vi "TCL Convert Datalog to CSV.vi"() -> ()   [LabVIEW 2010]
uses:
  <vilib>/Utility/file.llb/Write To Spreadsheet File (string).vi
panel:
  out "of":dbl
  out "file":i32
  out "file progress":dbl(slide) scale=0.0..1.0
  in  "primary key":string="EventNum"
  in  "signals":string[](array[string])=["RawSignal", "PolySignal"]
  out "error out":errorcluster
  in  "error in (no error)":errorcluster
  in  "input files (prompt)":path[](array[path])
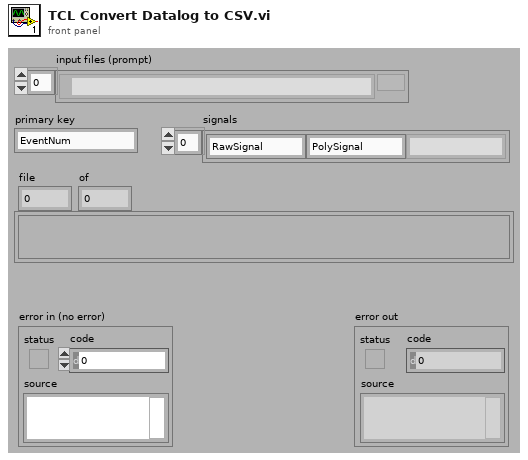
[diagram p1: front panel]
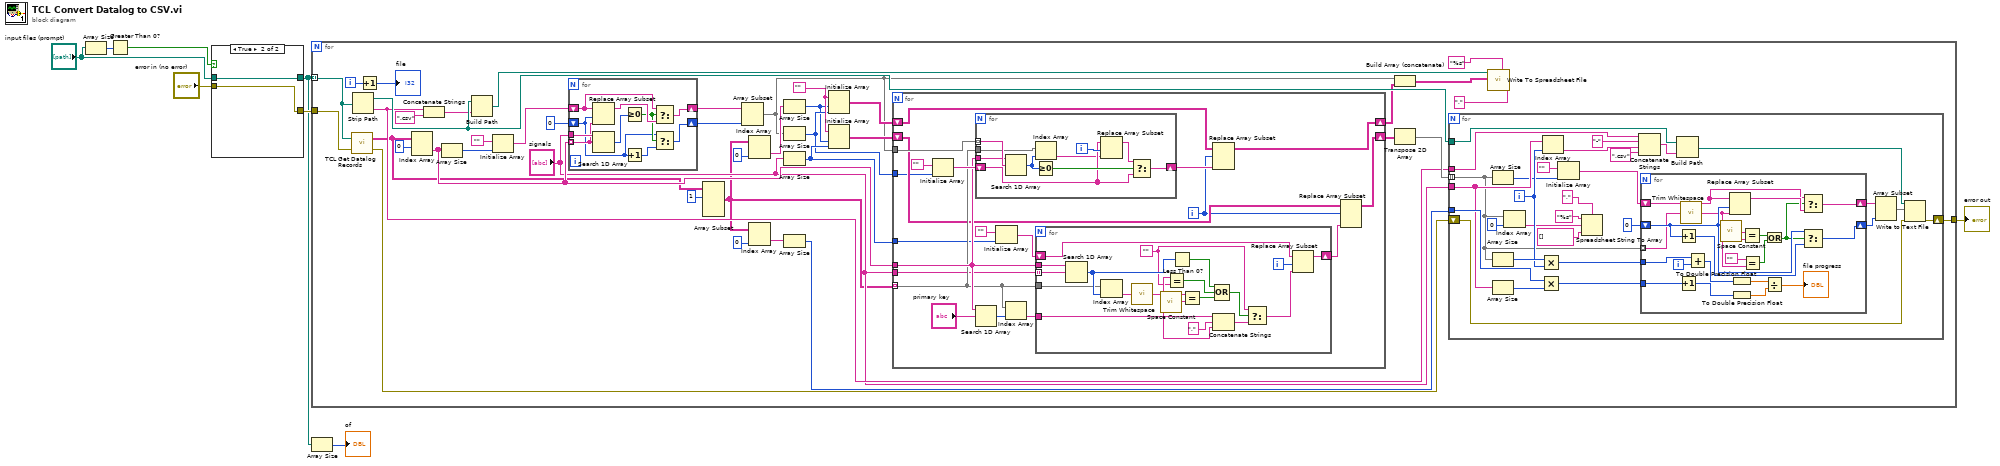
[diagram p0: block diagram]
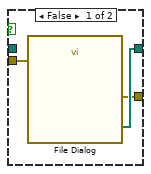
[diagram p2: hidden frame]
diagram:
  n1 = Array Size(array="input files (prompt)") -> (size(s)=w8:i32)
  n2 = Greater Than 0?(x=w8) -> (x > 0?=w7:bool)
  n3 = case shown="True" w7 {
    tunnel: [w11 w12] -> w2
    tunnel: "error in (no error)" -> [w10 w13]
    tunnel: [w9 w13] -> w5
    tunnel: "input files (prompt)" -> [_ w12]
    frame False {
      n4 = call "File Dialog"("error in"=w10) -> ("selected paths"=w11:path[], "error out"=w9:errorcluster)  [unwired: 11 in, 2 out]
    }
    frame True {
    }
  }
  n5 = for {
    tunnel: w2 -> [w50] mode=indexing
    tunnel: w5 -> [w42]
    tunnel: [w15] -> w3
    i -> [w34]
    w21 = ""
    n6 = call "TCL Get Datalog Records.vi"("error in (no error)"=w42, "event file"=w50) -> ("error out"=w14:errorcluster, "records"=w16:string[][])
    n7 = Strip Path(path=w50) -> (stripped path=w49:path, name=w46:string)
    n8 = Increment(x=w34) -> (x+1=→"file":i32)
    n9 = Index Array(array=w16, index (row)=0) -> (element=w31:string[])  [unwired: 1 in]
    n10 = Concatenate Strings(w46, ".csv" ("string")) -> (w48:string)
    n11 = Array Size(array=w31) -> (size(s)=w32:i32)
    n12 = Build Path(base path=w49, name or relative path=w48) -> (appended path=w43:path)
    n13 = Initialize Array("", w32) -> (w29:string[])
    n14 = for {
      tunnel: w31 -> [w159] mode=indexing
      tunnel: "signals" -> [w163]
      shift-right: [w161] -> w37
      shift-left: w29 -> [w158]
      shift-right: [w157] -> w28
      shift-left: 0 -> [w154]
      n15 = Replace Array Subset(array=w158, new element=w159, index=w154) -> (w160:string[])
      n16 = Search 1D Array(1D array=w163, element=w159) -> (index of element=w162:i32)  [unwired: 1 in]
      n17 = Greater Or Equal To 0?(x=w162) -> (x >= 0?=w156:bool)
      n18 = Increment(x=w154) -> (x+1=w155:i32)
      n19 = Select(t=w158, s=w156, f=w160) -> (s? t:f=w161:string[])
      n20 = Select(t=w154, s=w156, f=w155) -> (s? t:f=w157:i32)
    }
    n21 = Array Subset(array=w16, index (row)=1 ("index")) -> (w24:string[][])  [unwired: 3 in]
    n22 = Array Subset(array=w37, length=w28) -> (w20:string[])  [unwired: 1 in]
    n23 = Index Array(array=w24, index (col)=0 ("index (row)")) -> (element=w23:string[])  [unwired: 1 in]
    n24 = Index Array(array=w24, index (col)=0 ("disabled index (col)")) -> (element=w40:string[])  [unwired: 1 in]
    n25 = Array Size(array=w23) -> (size(s)=w18:i32)
    n26 = Array Size(array=w20) -> (size(s)=w19:i32)
    n27 = Array Size(array="signals") -> (size(s)=w25:i32)
    n28 = Array Size(array=w40) -> (size(s)=w36:i32)
    n29 = Initialize Array(w21, w18, w19) -> (w22:string[][])
    n30 = Initialize Array(w21, w18, w25) -> (w27:string[][])
    n31 = for {
      tunnel: w24 -> [w119] mode=indexing
      tunnel: w20 -> [w124]
      tunnel: w31 -> [w121]
      tunnel: "signals" -> [w111]
      shift-right: [w116] -> w52
      shift-left: w27 -> [w115]
      shift-right: [w113] -> w38
      shift-left: w22 -> [w114]
      tunnel: w25 -> [w109]
      tunnel: w19 -> [w108]
      i -> [w105]
      n32 = Initialize Array("", w108) -> (w122:string[])
      n33 = for {
        tunnel: w124 -> [w153] mode=indexing
        tunnel: w121 -> [w152]
        shift-right: [w150] -> w107
        shift-left: w122 -> [w146]
        tunnel: w119 -> [w149]
        i -> [w147]
        n34 = Search 1D Array(1D array=w152, element=w153) -> (index of element=w148:i32)  [unwired: 1 in]
        n35 = Greater Or Equal To 0?(x=w148) -> (x >= 0?=w151:bool)
        n36 = Index Array(array=w149, index=w148) -> (element=w145:string)
        n37 = Replace Array Subset(array=w146, new element=w145, index=w147) -> (w144:string[])
        n38 = Select(t=w144, s=w151, f=w146) -> (s? t:f=w150:string[])
      }
      n39 = Search 1D Array(1D array=w121, element="primary key") -> (index of element=w118:i32)  [unwired: 1 in]
      n40 = Initialize Array("", w109) -> (w112:string[])
      n41 = Index Array(array=w119, index=w118) -> (element=w117:string)
      n42 = for {
        tunnel: w111 -> [w142] mode=indexing
        tunnel: w121 -> [w143]
        shift-right: [w136] -> w106
        shift-left: w112 -> [w139]
        tunnel: w119 -> [w140]
        tunnel: w117 -> [w138]
        i -> [w135]
        w127 = ""
        n43 = Search 1D Array(1D array=w143, element=w142) -> (index of element=w141:i32)  [unwired: 1 in]
        n44 = Index Array(array=w140, index=w141) -> (element=w131:string)
        n45 = call <vilib>:"Trim Whitespace.vi"("string"=w131) -> ("trimmed string"=w129:string)  [unwired: 1 in]
        n46 = call <vilib>:"Space Constant.vi"() -> ("String"=w130:string)
        n47 = Equal?(x=w129, y=w127) -> (x = y?=w133:bool)
        n48 = Less Than 0?(x=w141) -> (x < 0?=w126:bool)
        n49 = Equal?(x=w129, y=w130) -> (x = y?=w132:bool)
        n50 = Concatenate Strings(w138, "," ("string"), w129) -> (w128:string)
        n51 = Compound Arithmetic op=OR(w126, w133, w132) -> (w125:bool)
        n52 = Select(t=w127, s=w125, f=w128) -> (s? t:f=w134:string)
        n53 = Replace Array Subset(array=w139, new element=w134, index=w135) -> (w136:string[])
      }
      n54 = Replace Array Subset(array=w114, new element=w107, index (row)=w105) -> (w113:string[][])  [unwired: 1 in]
      n55 = Replace Array Subset(array=w115, new element=w106, index (row)=w105) -> (w116:string[][])  [unwired: 1 in]
    }
    n56 = Build Array (concatenate)(w20, w38) -> (w39:string[][])
    n57 = Transpose 2D Array(2D array=w52) -> (transposed array=w51:string[][])
    n58 = for {
      tunnel: w51 -> [w63] mode=indexing
      tunnel: w49 -> [w83]
      tunnel: w46 -> [w81]
      tunnel: "signals" -> [w72]
      tunnel: w36 -> [w73]
      shift-right: [w56] -> w15
      shift-left: w14 -> [w55]
      i -> [w76]
      n59 = Array Size(array=w63) -> (size(s)=w62:i32)
      n60 = Array Size(array=w63) -> (size(s)=w77:i32)
      n61 = Array Size(array=w72) -> (size(s)=w71:i32)
      n62 = Index Array(array=w63, index=0) -> (element=w68:string)
      n63 = Multiply(x=w77, y=w76) -> (x*y=w75:i32)
      n64 = Multiply(x=w73, y=w71) -> (x*y=w74:i32)
      n65 = Index Array(array=w72, index=w76) -> (element=w79:string)
      n66 = Initialize Array("", w62) -> (w64:string[])
      n67 = Spreadsheet String To Array(delimiter (Tab)=",", format string="%s", spreadsheet string=w68, array type (2D Dbl)=string[] []) -> ()  [unwired: 1 out]
      n68 = Concatenate Strings(w81, "-" ("string"), w79, ".csv" ("string")) -> (w82:string)
      n69 = for {
        tunnel: w63 -> [w87] mode=indexing
        shift-right: [w98] -> w59
        shift-left: w64 -> [w96]
        tunnel: w74 -> [w102]
        tunnel: w75 -> [w100]
        shift-right: [w94] -> w60
        shift-left: 0 -> [w93]
        i -> [w99]
        n70 = Increment(x=w93) -> (x+1=w92:i32)
        n71 = Increment(x=w102) -> (x+1=w91:i32)
        n72 = call <vilib>:"Trim Whitespace.vi"("string"=w87) -> ("trimmed string"=w85:string)  [unwired: 1 in]
        n73 = Add(x=w100, y=w99) -> (x+y=w101:i32)
        n74 = call <vilib>:"Space Constant.vi"() -> ("String"=w90:string)
        n75 = Replace Array Subset(array=w96, new element=w85, index=w93) -> (w97:string[])
        n76 = To Double Precision Float(number=w101) -> (double precision float=w103:dbl)
        n77 = To Double Precision Float(number=w91) -> (double precision float=w104:dbl)
        n78 = Equal?(x=w90, y=w85) -> (x = y?=w95:bool)
        n79 = Equal?(x="", y=w85) -> (x = y?=w88:bool)
        n80 = Or(x=w95, y=w88) -> (x .or. y?=w89:bool)
        n81 = Divide(x=w103, y=w104) -> (x/y=→"file progress":dbl)
        n82 = Select(t=w96, s=w89, f=w97) -> (s? t:f=w98:string[])
        n83 = Select(t=w93, s=w89, f=w92) -> (s? t:f=w94:i32)
      }
      n84 = Build Path(base path=w83, name or relative path=w82) -> (appended path=w58:path)
      n85 = Array Subset(array=w59, length=w60) -> (w57:string[])  [unwired: 1 in]
      n86 = Write to Text File(file (use dialog)=w58, text=w57, error in=w55) -> (error out=w56:errorcluster)  [unwired: 1 in, 2 out]
    }
    n87 = call-poly <vilib>:"Write To Spreadsheet File.vi"("delimiter (\\t)"="," ("delimiter (\\t)"), "format (%s)"="%s" ("format (%.3f)"), "2D data"=w39, "file path (dialog if empty)"=w43) -> ()  [unwired: 4 in, 1 out]
  }
  "error out" <- w3
  n88 = Array Size(array=w2) -> (size(s)=→"of":i32)
